vi "SE Initialization VI.vi"(8 "error in (no error)":errorcluster, 10 "Custom XML":string, 11 "Device Item Ref in":T1 format="%.0x") -> (0 "error out":errorcluster, 3 "Device Item Ref out":T1 format="%.0x")   [LabVIEW 2011, in "Chassis TimeSync System Explorer.lvlib"]
uses:
  Chassis TimeSync System Explorer.lvlib
  <vilib>/NI Veristand/Custom Device API/Custom Device Item Ref.ctl
  <vilib>/NI Veristand/Custom Device API/Custom Device Channel Type.ctl
  Shared/Constants.vi
  <vilib>/NI Veristand/Custom Device API/Custom Device API.lvlib
  Shared/Chassis TimeSync Shared.lvlib
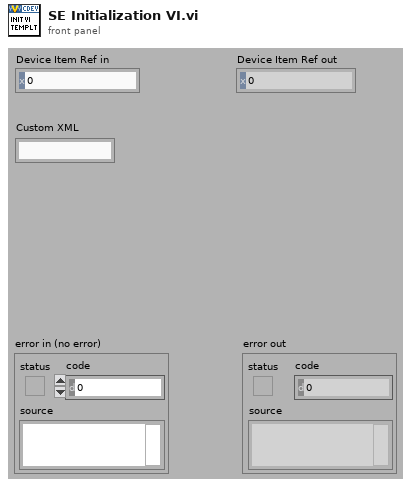
[diagram p1: front panel]
types:
  T1 = typedef "Custom Device API.lvlib/Custom Device Item Ref.ctl" = u64
  T2 = typedef "Custom Device API.lvlib/Custom Device Channel Type.ctl" = enum16{"Input", "Output"}
  T3 = typedef "Chassis TimeSync Shared.lvlib/Channel.ctl" = cluster{"Name":string, "Units":string, "Default":dbl, "Description":string}
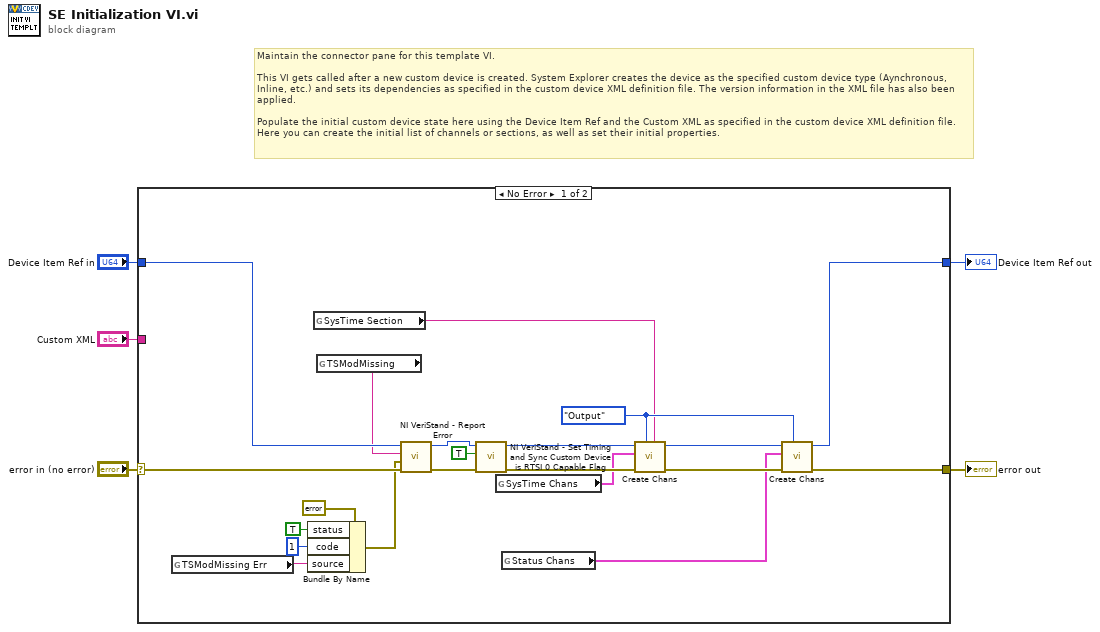
[diagram p0: block diagram]
diagram:
  # "Maintain the connector pane for this template VI.\n\nThis VI gets called after a new custom device is created. System Explorer creates the device as the specified custom device type (Aynchronous, Inline, etc.) and sets its dependencies as specified in the custom device XML definition file. The version information in the XML file has also been applied.\n\nPopulate the initial custom device state here using the Device Item Ref and the Custom XML as specified in the custom device XML definition file. Here you can create the initial list of channels or sections, as well as set their initial properties."
  n1 = case shown="No Error" "error in (no error)" {
    selector: "error in (no error)" -> [w17 w28]
    tunnel: [w10 w28] -> w5
    tunnel: [w9 w27] -> w3
    tunnel: "Device Item Ref in" -> [w19 w27]
    tunnel: "Custom XML" -> [_ _]
    frame No Error {
      w7 = Custom_Device_Channel_Type."Output" ("Type")
      n2 = global read "Constants.vi" "TSModMissing Err"() -> (w12:string)
      n3 = Bundle By Name(cluster=errorcluster {"status"=FALSE, "code"=0, "source"=""} ("error constant"), "status"=TRUE, "code"=1, "source"=w12) -> (w11:errorcluster)
      n4 = global read "Constants.vi" "SysTime Section"() -> (w6:string)
      n5 = global read "Constants.vi" "TSModMissing"() -> (w16:string)
      n6 = call <vilib>:"NI VeriStand - Report Error.vi"("error in (no error)"=w17, "New Error"=w11, "Error ID"=w16, "Node Ref in"=w19) -> ("error out"=w20:errorcluster, "Node Ref out"=w18:T1)  [unwired: 6 in]
      n7 = call <vilib>:"NI VeriStand - Set Timing and Sync Custom Device is RTSI 0 Capable Flag.vi"("error in (no error)"=w20, "Is RTSI 0 Capable"=TRUE, "Device Ref in"=w18) -> ("error out"=w25:errorcluster, "Device Ref out"=w24:T1)  [unwired: 7 in]
      n8 = global read "Constants.vi" "SysTime Chans"() -> (w23:T3[])
      n9 = global read "Constants.vi" "Status Chans"() -> (w8:T3[])
      n10 = call "Create Chans.vi"("New Section Name (none)"=w6, "Type"=w7, "error in (no error)"=w25, "Channels"=w23, "Section Ptr"=w24) -> ("error out"=w22:errorcluster, "Section Ptr dup"=w21:T1)  [unwired: 5 in]
      n11 = call "Create Chans.vi"("Type"=w7, "error in (no error)"=w22, "Channels"=w8, "Section Ptr"=w21) -> ("error out"=w10:errorcluster, "Section Ptr dup"=w9:T1)  [unwired: 6 in]
    }
    frame Error {
    }
  }
  "error out" <- w5
  "Device Item Ref out" <- w3
